vi "ALTS-2015 Decide Cases to go.vi"(8 "error in":errorcluster, 11 "DI Change Status":bool[](array[boolean])) -> (0 "error out":errorcluster, 2 "Station Selected":T1[](array[typedef]), 3 "Cases to go":string)   [LabVIEW 2013]
doc: "Copyright © 2005, Soliton Technologies.\nAll rights reserved."
uses:
  Controls/ALTS-2015 Station Cluster.ctl
  Controls/ALTS-2015 LV2GBL Options.ctl
  SLL DAQ Engine/Software/Source Code/Sub VIs/DAQ Engine/Controls/SLL DE List of Digital Inputs.ctl
  Controls/ALTS-2015 States.ctl
  Controls/ALTS-2015 Air Leak Test System-Main Screen Cases.ctl
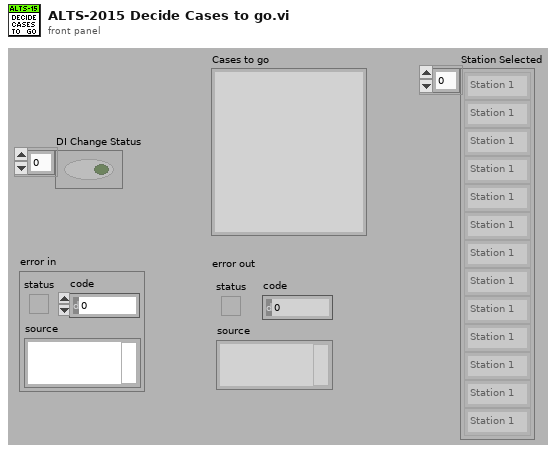
[diagram p1: front panel]
types:
  T1 = typedef "ALTS-2015 Station Cluster.ctl" = enum16{"Station 1", "Station 2", "Station 3", "Station 4"}
  T2 = typedef "ALTS-2015 LV2GBL Options.ctl" = enum16{"Read all", "Write all"}
  T3 = typedef "SLL DE List of Digital Inputs.ctl" = enum16{"STATION1_START", "STATION1_STOP", "STATION1_CLAMPED", "STATION1_TC_PASS", "STATION1_TC_FAIL", "STATION2_START", "STATION2_STOP", "STATION2_CLAMPED", "STATION2_TC_PASS", "STATION2_TC_FAIL", "STATION3_START", "STATION3_STOP", "STATION3_CLAMPED", "STATION3_TC_PASS", "STATION3_TC_FAIL", "STATION4_START", "STATION4_STOP", "STATION4_CLAMPED", "STATION4_TC_PASS", "STATION4_TC_FAIL"}
  T4 = typedef "ALTS-2015 Air Leak Test System-Main Screen Cases.ctl" = enum16{">PollEvents", ">Initialize", ">Exit", ">Error", ">EmptyCase", ">Get User Login", ">Initial FP update", ">Scan Serial Number", ">Check DI Status", ">Check for UUT Clamped & start Test", ">Stop the Test", ">Restore station after stop pressed", ">UUT Clamped", ">UUT Unclamped", ">Test Complete Failed", ">Read Test Data Result - Pass", ">Read Test Data Result - Fail", ">Write Result to DB", ">Update Station Info"}
  T5 = typedef "ALTS-2015 States.ctl" = enum16{"Initialize", "Poll", "Error", "Exit", "Authentication", "Scan Serial No", "Enqueue New Serial Task", "Enqueue Invalid Serial Task", "Enqueue Rerun Task", "Enqueu Unload Task", "Check DI Status", "Check UUT Clamp & Start Test", "Restore station after Stop Pressed", "Stop the Test", "UUT Clamped", "UUT Unclamped", "Test Complete Failed", "Read Test Data Result - Pass", "Read Test Data Result - Fail", "Write Result to DB", "Update Station Info"}
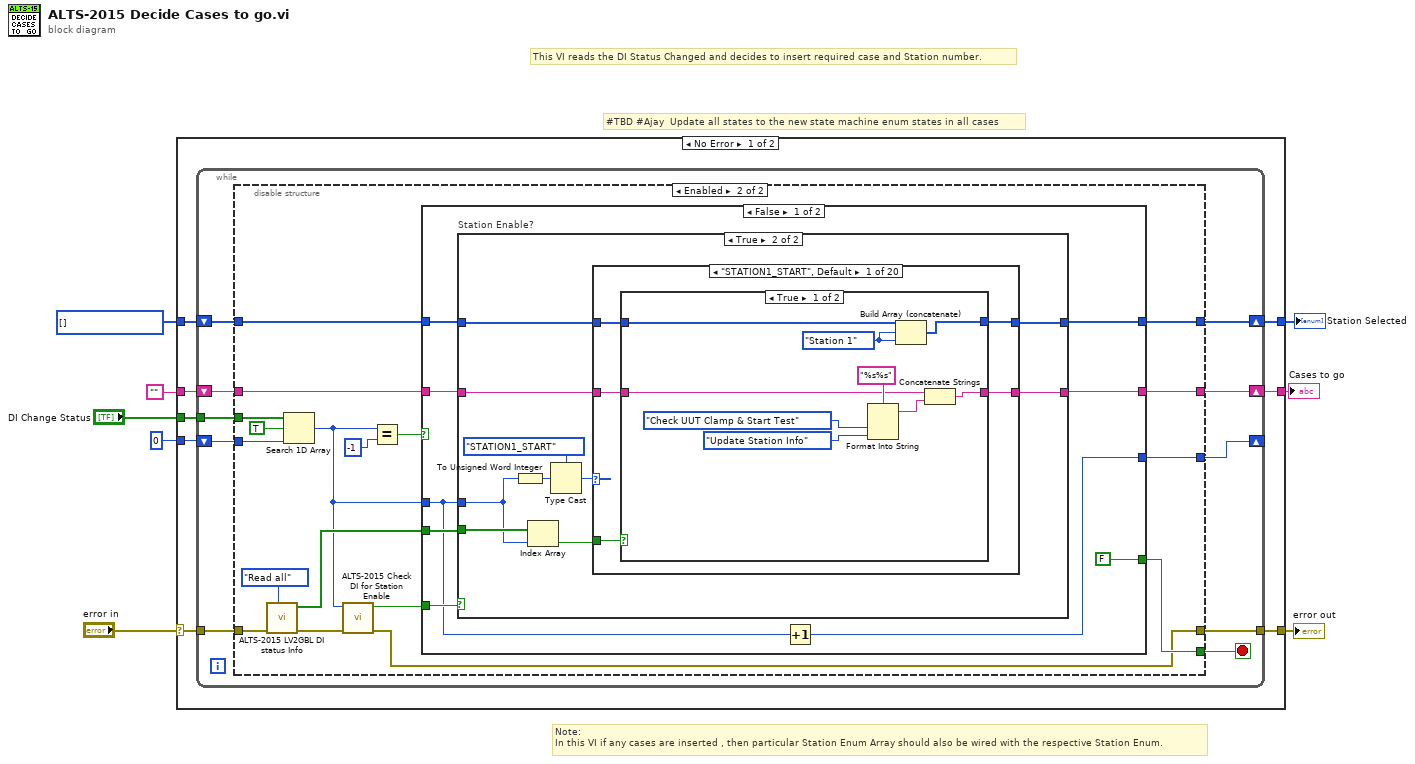
[diagram p0: block diagram]
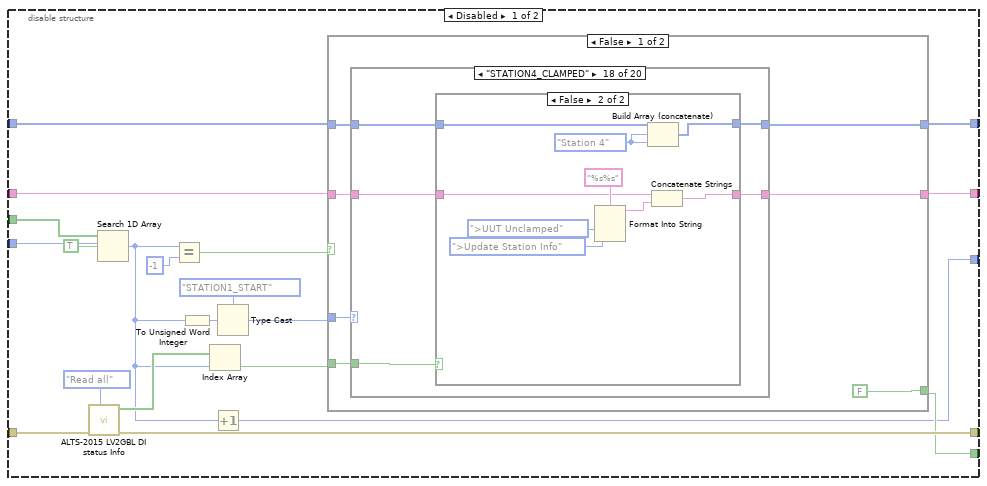
[diagram p2: hidden frame]
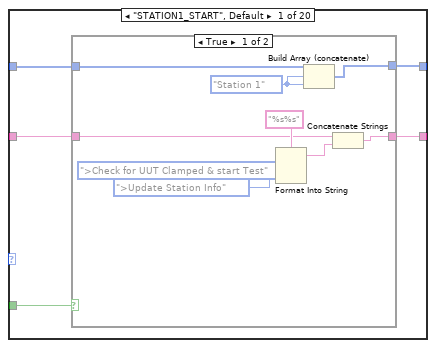
[diagram p3: hidden frame]
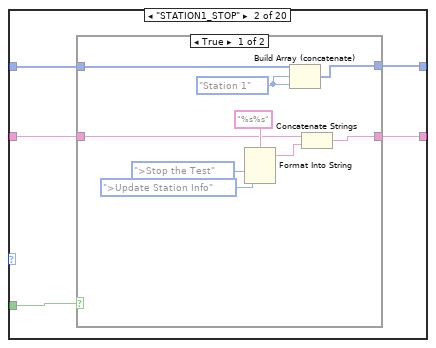
[diagram p5: hidden frame]
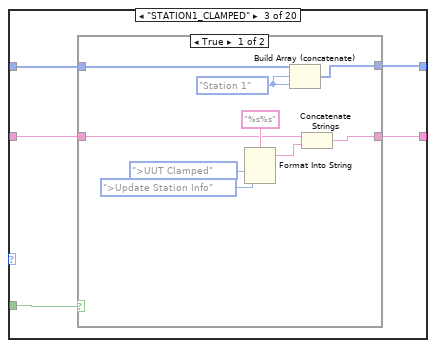
[diagram p7: hidden frame]
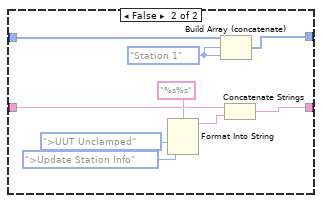
[diagram p8: hidden frame]
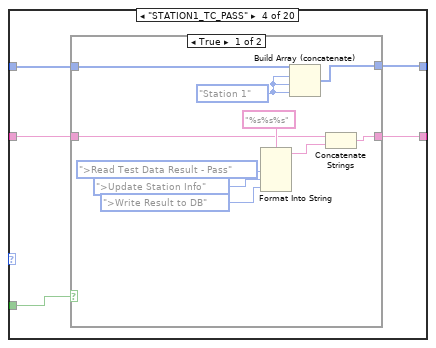
[diagram p9: hidden frame]
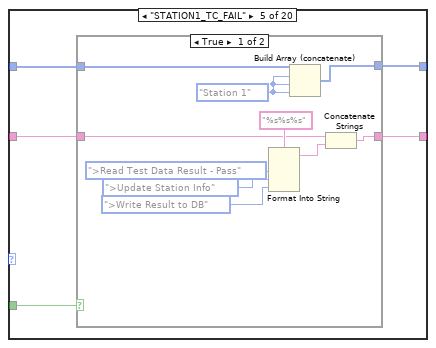
[diagram p11: hidden frame]
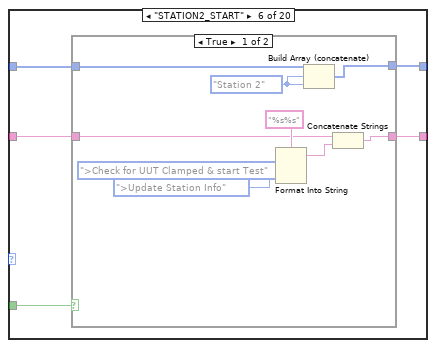
[diagram p13: hidden frame]
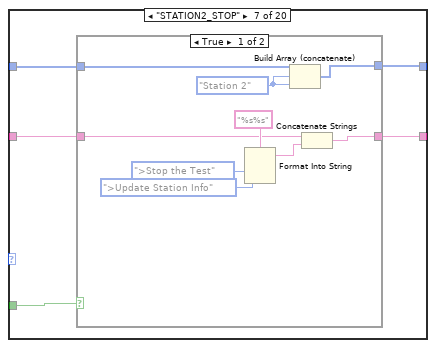
[diagram p15: hidden frame]
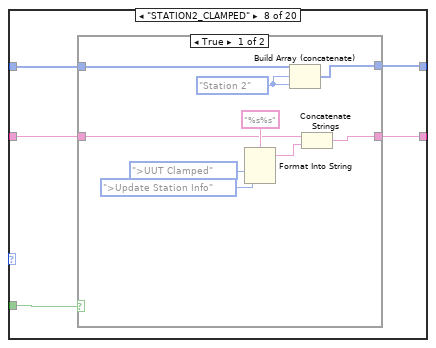
[diagram p17: hidden frame]
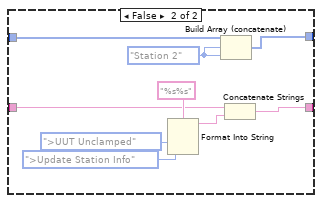
[diagram p18: hidden frame]
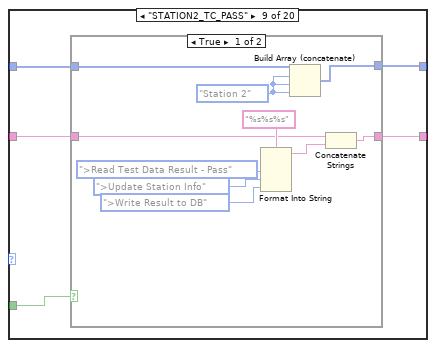
[diagram p19: hidden frame]
diagram:
  w3 = T1[] [] items=["Station 1", "Station 2", "Station 3", "Station 4"]
  # "#TBD #Ajay  Update all states to the new state machine enum states in all cases"
  # "Note: \nIn this VI if any cases are inserted , then particular Station Enum Array should also be wired with the respective Station Enum."
  # "This VI reads the DI Status Changed and decides to insert required case and Station number."
  n1 = case shown="No Error" "error in" {
    selector: "error in" -> [w14 w802]
    tunnel: [w13 w802] -> w8
    tunnel: "DI Change Status" -> [w10 _]
    tunnel: "" -> [w16 _]
    tunnel: [w15 ""] -> w4
    tunnel: w3 -> [w12 _]
    tunnel: [w11 w800] -> w2
    tunnel: 0 ("index of element") -> [w9 _]
    frame No Error {
      n2 = while {
        shift-right: [w20] -> w15
        shift-left: w16 -> [w26]
        tunnel: w14 -> [w25]
        tunnel: [w24] -> w13
        shift-right: [w22] -> w11
        shift-left: w12 -> [w23]
        tunnel: w10 -> [w19]
        shift-right: [w17] -> _
        shift-left: w9 -> [w18]
        stop <- w21 stop-if-true
        n3 = disable-structure shown="Enabled" {
          disable-tunnel: w26 -> [w41 w428]
          disable-tunnel: w25 -> [w39 w426]
          disable-tunnel: [w36 w413] -> w24
          disable-tunnel: w23 -> [w35 w424]
          disable-tunnel: [w34 w423] -> w22
          disable-tunnel: [w32 w422] -> w21
          disable-tunnel: [w31 w421] -> w20
          disable-tunnel: w19 -> [w30 w420]
          disable-tunnel: w18 -> [w28 w419]
          disable-tunnel: [w27 w418] -> w17
          frame Disabled {
            n4 = call "ALTS-2015 LV2GBL DI status Info.vi"("Options"=ALTS-2015_LV2GBL_Options."Read all", "error in"=w39) -> ("error out"=w36:errorcluster, "DI Status Out"=w38:bool[])  [unwired: 8 in]
            n5 = Search 1D Array(1D array=w30, element=TRUE, start index (0)=w28) -> (index of element=w29:i32)
            n6 = Equal?(x=w29, y=-1) -> (x = y?=w33:bool)
            n7 = To Unsigned Word Integer(number=w29) -> (unsigned 16bit integer=w43:u16)
            n8 = Index Array(array=w38, index=w29) -> (element=w37:bool)
            n9 = Increment(x=w29) -> (x+1=w27:i32)
            n10 = Type Cast(type=SLL_DE_List_of_Digital_Inputs."STATION1_START" ("DI Channel Name"), x=w43) -> (*(type *) &x=w42:T3)
            n11 = case shown="False" w33 {
              tunnel: w42 -> [w53 _]
              tunnel: w41 -> [w48 w411]
              tunnel: w37 -> [w52 _]
              tunnel: w35 -> [w51 w410]
              tunnel: [w50 w410] -> w34
              tunnel: [FALSE TRUE] -> w32
              tunnel: [w47 w411] -> w31
              frame False {
                n12 = case shown="\"STATION4_CLAMPED\"" w53 {
                  tunnel: w52 -> [w58 w74 w90 w113 w130 w147 w163 w179 w202 w219 w236 w252 w268 w291 w308 w325 w341 w357 w380 w397]
                  tunnel: w51 -> [w57 w73 w89 w112 w129 w146 w162 w178 w201 w218 w235 w251 w267 w290 w307 w324 w340 w356 w379 w396]
                  tunnel: [w56 w72 w88 w111 w128 w145 w161 w177 w200 w217 w234 w250 w266 w289 w306 w323 w339 w355 w378 w395] -> w50
                  tunnel: w48 -> [w55 w71 w87 w110 w127 w144 w160 w176 w199 w216 w233 w249 w265 w288 w305 w322 w338 w354 w377 w394]
                  tunnel: [w54 w70 w86 w109 w126 w143 w159 w175 w198 w215 w232 w248 w264 w287 w304 w321 w337 w353 w376 w393] -> w47
                  frame "STATION1_START", Default {
                    n13 = case shown="True" w58 {
                      tunnel: w57 -> [w65 w69]
                      tunnel: [w64 w69] -> w56
                      tunnel: w55 -> [w63 w68]
                      tunnel: [w61 w68] -> w54
                      frame True {
                        w59 = ALTS-2015_Station_Cluster."Station 1" ("Station Cluster")
                        n14 = Format Into String(format string="%s%s", ALTS-2015_Air_Leak_Test_System-Main_Screen_Cases.">Check for UUT Clamped & start Test" ("Cases"), ALTS-2015_Air_Leak_Test_System-Main_Screen_Cases.">Update Station Info" ("input 2")) -> (resulting string=w62:string)  [unwired: 2 in, 1 out]
                        n15 = Build Array (concatenate)(w65, w59, w59) -> (w64:T1[])
                        n16 = Concatenate Strings(w63, w62) -> (w61:string)
                      }
                      frame False {
                      }
                    }
                  }
                  frame "STATION1_STOP" {
                    n17 = case shown="True" w74 {
                      tunnel: w73 -> [w81 w85]
                      tunnel: [w80 w85] -> w72
                      tunnel: w71 -> [w79 w84]
                      tunnel: [w77 w84] -> w70
                      frame True {
                        w75 = ALTS-2015_Station_Cluster."Station 1" ("Station Cluster")
                        n18 = Format Into String(format string="%s%s", ALTS-2015_Air_Leak_Test_System-Main_Screen_Cases.">Stop the Test" ("Cases"), ALTS-2015_Air_Leak_Test_System-Main_Screen_Cases.">Update Station Info" ("input 2")) -> (resulting string=w78:string)  [unwired: 2 in, 1 out]
                        n19 = Build Array (concatenate)(w81, w75, w75) -> (w80:T1[])
                        n20 = Concatenate Strings(w79, w78) -> (w77:string)
                      }
                      frame False {
                      }
                    }
                  }
                  frame "STATION1_CLAMPED" {
                    n21 = case shown="True" w90 {
                      tunnel: w89 -> [w97 w106]
                      tunnel: [w96 w105] -> w88
                      tunnel: w87 -> [w95 w104]
                      tunnel: [w93 w102] -> w86
                      frame True {
                        w91 = ALTS-2015_Station_Cluster."Station 1" ("Station Cluster")
                        n22 = Format Into String(format string="%s%s", ALTS-2015_Air_Leak_Test_System-Main_Screen_Cases.">UUT Clamped" ("Cases"), ALTS-2015_Air_Leak_Test_System-Main_Screen_Cases.">Update Station Info" ("input 2")) -> (resulting string=w94:string)  [unwired: 2 in, 1 out]
                        n23 = Build Array (concatenate)(w97, w91, w91) -> (w96:T1[])
                        n24 = Concatenate Strings(w95, w94) -> (w93:string)
                      }
                      frame False {
                        w100 = ALTS-2015_Station_Cluster."Station 1" ("Station Cluster")
                        n25 = Format Into String(format string="%s%s", ALTS-2015_Air_Leak_Test_System-Main_Screen_Cases.">UUT Unclamped" ("Cases"), ALTS-2015_Air_Leak_Test_System-Main_Screen_Cases.">Update Station Info" ("input 2")) -> (resulting string=w103:string)  [unwired: 2 in, 1 out]
                        n26 = Build Array (concatenate)(w106, w100, w100) -> (w105:T1[])
                        n27 = Concatenate Strings(w104, w103) -> (w102:string)
                      }
                    }
                  }
                  frame "STATION1_TC_PASS" {
                    n28 = case shown="True" w113 {
                      tunnel: w112 -> [w121 w125]
                      tunnel: [w120 w125] -> w111
                      tunnel: w110 -> [w119 w124]
                      tunnel: [w117 w124] -> w109
                      frame True {
                        w114 = ALTS-2015_Station_Cluster."Station 1" ("Station Cluster")
                        n29 = Format Into String(format string="%s%s%s", ALTS-2015_Air_Leak_Test_System-Main_Screen_Cases.">Read Test Data Result - Pass" ("Cases"), ALTS-2015_Air_Leak_Test_System-Main_Screen_Cases.">Update Station Info" ("input 2"), ALTS-2015_Air_Leak_Test_System-Main_Screen_Cases.">Write Result to DB" ("input 2")) -> (resulting string=w118:string)  [unwired: 2 in, 1 out]
                        n30 = Build Array (concatenate)(w121, w114, w114, w114) -> (w120:T1[])
                        n31 = Concatenate Strings(w119, w118) -> (w117:string)
                      }
                      frame False {
                      }
                    }
                  }
                  frame "STATION1_TC_FAIL" {
                    n32 = case shown="True" w130 {
                      tunnel: w129 -> [w138 w142]
                      tunnel: [w137 w142] -> w128
                      tunnel: w127 -> [w136 w141]
                      tunnel: [w134 w141] -> w126
                      frame True {
                        w131 = ALTS-2015_Station_Cluster."Station 1" ("Station Cluster")
                        n33 = Format Into String(format string="%s%s%s", ALTS-2015_Air_Leak_Test_System-Main_Screen_Cases.">Read Test Data Result - Pass" ("Cases"), ALTS-2015_Air_Leak_Test_System-Main_Screen_Cases.">Update Station Info" ("input 2"), ALTS-2015_Air_Leak_Test_System-Main_Screen_Cases.">Write Result to DB" ("input 3")) -> (resulting string=w135:string)  [unwired: 2 in, 1 out]
                        n34 = Build Array (concatenate)(w138, w131, w131, w131) -> (w137:T1[])
                        n35 = Concatenate Strings(w136, w135) -> (w134:string)
                      }
                      frame False {
                      }
                    }
                  }
                  frame "STATION2_START" {
                    n36 = case shown="True" w147 {
                      tunnel: w146 -> [w154 w158]
                      tunnel: [w153 w158] -> w145
                      tunnel: w144 -> [w152 w157]
                      tunnel: [w150 w157] -> w143
                      frame True {
                        w148 = ALTS-2015_Station_Cluster."Station 2" ("Station Cluster")
                        n37 = Format Into String(format string="%s%s", ALTS-2015_Air_Leak_Test_System-Main_Screen_Cases.">Check for UUT Clamped & start Test" ("Cases"), ALTS-2015_Air_Leak_Test_System-Main_Screen_Cases.">Update Station Info" ("input 2")) -> (resulting string=w151:string)  [unwired: 2 in, 1 out]
                        n38 = Build Array (concatenate)(w154, w148, w148) -> (w153:T1[])
                        n39 = Concatenate Strings(w152, w151) -> (w150:string)
                      }
                      frame False {
                      }
                    }
                  }
                  frame "STATION2_STOP" {
                    n40 = case shown="True" w163 {
                      tunnel: w162 -> [w170 w174]
                      tunnel: [w169 w174] -> w161
                      tunnel: w160 -> [w168 w173]
                      tunnel: [w166 w173] -> w159
                      frame True {
                        w164 = ALTS-2015_Station_Cluster."Station 2" ("Station Cluster")
                        n41 = Format Into String(format string="%s%s", ALTS-2015_Air_Leak_Test_System-Main_Screen_Cases.">Stop the Test" ("Cases"), ALTS-2015_Air_Leak_Test_System-Main_Screen_Cases.">Update Station Info" ("input 2")) -> (resulting string=w167:string)  [unwired: 2 in, 1 out]
                        n42 = Build Array (concatenate)(w170, w164, w164) -> (w169:T1[])
                        n43 = Concatenate Strings(w168, w167) -> (w166:string)
                      }
                      frame False {
                      }
                    }
                  }
                  frame "STATION2_CLAMPED" {
                    n44 = case shown="True" w179 {
                      tunnel: w178 -> [w186 w195]
                      tunnel: [w185 w194] -> w177
                      tunnel: w176 -> [w184 w193]
                      tunnel: [w182 w191] -> w175
                      frame True {
                        w180 = ALTS-2015_Station_Cluster."Station 2" ("Station Cluster")
                        n45 = Format Into String(format string="%s%s", ALTS-2015_Air_Leak_Test_System-Main_Screen_Cases.">UUT Clamped" ("Cases"), ALTS-2015_Air_Leak_Test_System-Main_Screen_Cases.">Update Station Info" ("input 2")) -> (resulting string=w183:string)  [unwired: 2 in, 1 out]
                        n46 = Build Array (concatenate)(w186, w180, w180) -> (w185:T1[])
                        n47 = Concatenate Strings(w184, w183) -> (w182:string)
                      }
                      frame False {
                        w189 = ALTS-2015_Station_Cluster."Station 2" ("Station Cluster")
                        n48 = Format Into String(format string="%s%s", ALTS-2015_Air_Leak_Test_System-Main_Screen_Cases.">UUT Unclamped" ("Cases"), ALTS-2015_Air_Leak_Test_System-Main_Screen_Cases.">Update Station Info" ("input 2")) -> (resulting string=w192:string)  [unwired: 2 in, 1 out]
                        n49 = Build Array (concatenate)(w195, w189, w189) -> (w194:T1[])
                        n50 = Concatenate Strings(w193, w192) -> (w191:string)
                      }
                    }
                  }
                  frame "STATION2_TC_PASS" {
                    n51 = case shown="True" w202 {
                      tunnel: w201 -> [w210 w214]
                      tunnel: [w209 w214] -> w200
                      tunnel: w199 -> [w208 w213]
                      tunnel: [w206 w213] -> w198
                      frame True {
                        w203 = ALTS-2015_Station_Cluster."Station 2" ("Station Cluster")
                        n52 = Format Into String(format string="%s%s%s", ALTS-2015_Air_Leak_Test_System-Main_Screen_Cases.">Read Test Data Result - Pass" ("Cases"), ALTS-2015_Air_Leak_Test_System-Main_Screen_Cases.">Update Station Info" ("input 2"), ALTS-2015_Air_Leak_Test_System-Main_Screen_Cases.">Write Result to DB" ("input 2")) -> (resulting string=w207:string)  [unwired: 2 in, 1 out]
                        n53 = Build Array (concatenate)(w210, w203, w203, w203) -> (w209:T1[])
                        n54 = Concatenate Strings(w208, w207) -> (w206:string)
                      }
                      frame False {
                      }
                    }
                  }
                  frame "STATION2_TC_FAIL" {
                    n55 = case shown="True" w219 {
                      tunnel: w218 -> [w227 w231]
                      tunnel: [w226 w231] -> w217
                      tunnel: w216 -> [w225 w230]
                      tunnel: [w223 w230] -> w215
                      frame True {
                        w220 = ALTS-2015_Station_Cluster."Station 2" ("Station Cluster")
                        n56 = Format Into String(format string="%s%s%s", ALTS-2015_Air_Leak_Test_System-Main_Screen_Cases.">Read Test Data Result - Pass" ("Cases"), ALTS-2015_Air_Leak_Test_System-Main_Screen_Cases.">Update Station Info" ("input 2"), ALTS-2015_Air_Leak_Test_System-Main_Screen_Cases.">Write Result to DB" ("input 3")) -> (resulting string=w224:string)  [unwired: 2 in, 1 out]
                        n57 = Build Array (concatenate)(w227, w220, w220, w220) -> (w226:T1[])
                        n58 = Concatenate Strings(w225, w224) -> (w223:string)
                      }
                      frame False {
                      }
                    }
                  }
                  frame "STATION3_START" {
                    n59 = case shown="True" w236 {
                      tunnel: w235 -> [w243 w247]
                      tunnel: [w242 w247] -> w234
                      tunnel: w233 -> [w241 w246]
                      tunnel: [w239 w246] -> w232
                      frame True {
                        w237 = ALTS-2015_Station_Cluster."Station 3" ("Station Cluster")
                        n60 = Format Into String(format string="%s%s", ALTS-2015_Air_Leak_Test_System-Main_Screen_Cases.">Check for UUT Clamped & start Test" ("Cases"), ALTS-2015_Air_Leak_Test_System-Main_Screen_Cases.">Update Station Info" ("input 2")) -> (resulting string=w240:string)  [unwired: 2 in, 1 out]
                        n61 = Build Array (concatenate)(w243, w237, w237) -> (w242:T1[])
                        n62 = Concatenate Strings(w241, w240) -> (w239:string)
                      }
                      frame False {
                      }
                    }
                  }
                  frame "STATION3_STOP" {
                    n63 = case shown="True" w252 {
                      tunnel: w251 -> [w259 w263]
                      tunnel: [w258 w263] -> w250
                      tunnel: w249 -> [w257 w262]
                      tunnel: [w255 w262] -> w248
                      frame True {
                        w253 = ALTS-2015_Station_Cluster."Station 3" ("Station Cluster")
                        n64 = Format Into String(format string="%s%s", ALTS-2015_Air_Leak_Test_System-Main_Screen_Cases.">Stop the Test" ("Cases"), ALTS-2015_Air_Leak_Test_System-Main_Screen_Cases.">Update Station Info" ("input 2")) -> (resulting string=w256:string)  [unwired: 2 in, 1 out]
                        n65 = Build Array (concatenate)(w259, w253, w253) -> (w258:T1[])
                        n66 = Concatenate Strings(w257, w256) -> (w255:string)
                      }
                      frame False {
                      }
                    }
                  }
                  frame "STATION3_CLAMPED" {
                    n67 = case shown="False" w268 {
                      tunnel: w267 -> [w275 w284]
                      tunnel: [w274 w283] -> w266
                      tunnel: w265 -> [w273 w282]
                      tunnel: [w271 w280] -> w264
                      frame True {
                        w269 = ALTS-2015_Station_Cluster."Station 3" ("Station Cluster")
                        n68 = Format Into String(format string="%s%s", ALTS-2015_Air_Leak_Test_System-Main_Screen_Cases.">UUT Clamped" ("Cases"), ALTS-2015_Air_Leak_Test_System-Main_Screen_Cases.">Update Station Info" ("input 2")) -> (resulting string=w272:string)  [unwired: 2 in, 1 out]
                        n69 = Build Array (concatenate)(w275, w269, w269) -> (w274:T1[])
                        n70 = Concatenate Strings(w273, w272) -> (w271:string)
                      }
                      frame False {
                        w278 = ALTS-2015_Station_Cluster."Station 3" ("Station Cluster")
                        n71 = Format Into String(format string="%s%s", ALTS-2015_Air_Leak_Test_System-Main_Screen_Cases.">UUT Unclamped" ("Cases"), ALTS-2015_Air_Leak_Test_System-Main_Screen_Cases.">Update Station Info" ("input 2")) -> (resulting string=w281:string)  [unwired: 2 in, 1 out]
                        n72 = Build Array (concatenate)(w284, w278, w278) -> (w283:T1[])
                        n73 = Concatenate Strings(w282, w281) -> (w280:string)
                      }
                    }
                  }
                  frame "STATION3_TC_PASS" {
                    n74 = case shown="True" w291 {
                      tunnel: w290 -> [w299 w303]
                      tunnel: [w298 w303] -> w289
                      tunnel: w288 -> [w297 w302]
                      tunnel: [w295 w302] -> w287
                      frame True {
                        w292 = ALTS-2015_Station_Cluster."Station 3" ("Station Cluster")
                        n75 = Format Into String(format string="%s%s%s", ALTS-2015_Air_Leak_Test_System-Main_Screen_Cases.">Read Test Data Result - Pass" ("Cases"), ALTS-2015_Air_Leak_Test_System-Main_Screen_Cases.">Update Station Info" ("input 2"), ALTS-2015_Air_Leak_Test_System-Main_Screen_Cases.">Write Result to DB" ("input 2")) -> (resulting string=w296:string)  [unwired: 2 in, 1 out]
                        n76 = Build Array (concatenate)(w299, w292, w292, w292) -> (w298:T1[])
                        n77 = Concatenate Strings(w297, w296) -> (w295:string)
                      }
                      frame False {
                      }
                    }
                  }
                  frame "STATION3_TC_FAIL" {
                    n78 = case shown="True" w308 {
                      tunnel: w307 -> [w316 w320]
                      tunnel: [w315 w320] -> w306
                      tunnel: w305 -> [w314 w319]
                      tunnel: [w312 w319] -> w304
                      frame True {
                        w309 = ALTS-2015_Station_Cluster."Station 3" ("Station Cluster")
                        n79 = Format Into String(format string="%s%s%s", ALTS-2015_Air_Leak_Test_System-Main_Screen_Cases.">Read Test Data Result - Pass" ("Cases"), ALTS-2015_Air_Leak_Test_System-Main_Screen_Cases.">Update Station Info" ("input 2"), ALTS-2015_Air_Leak_Test_System-Main_Screen_Cases.">Write Result to DB" ("input 3")) -> (resulting string=w313:string)  [unwired: 2 in, 1 out]
                        n80 = Build Array (concatenate)(w316, w309, w309, w309) -> (w315:T1[])
                        n81 = Concatenate Strings(w314, w313) -> (w312:string)
                      }
                      frame False {
                      }
                    }
                  }
                  frame "STATION4_START" {
                    n82 = case shown="True" w325 {
                      tunnel: w324 -> [w332 w336]
                      tunnel: [w331 w336] -> w323
                      tunnel: w322 -> [w330 w335]
                      tunnel: [w328 w335] -> w321
                      frame True {
                        w326 = ALTS-2015_Station_Cluster."Station 4" ("Station Cluster")
                        n83 = Format Into String(format string="%s%s", ALTS-2015_Air_Leak_Test_System-Main_Screen_Cases.">Check for UUT Clamped & start Test" ("Cases"), ALTS-2015_Air_Leak_Test_System-Main_Screen_Cases.">Update Station Info" ("input 2")) -> (resulting string=w329:string)  [unwired: 2 in, 1 out]
                        n84 = Build Array (concatenate)(w332, w326, w326) -> (w331:T1[])
                        n85 = Concatenate Strings(w330, w329) -> (w328:string)
                      }
                      frame False {
                      }
                    }
                  }
                  frame "STATION4_STOP" {
                    n86 = case shown="True" w341 {
                      tunnel: w340 -> [w348 w352]
                      tunnel: [w347 w352] -> w339
                      tunnel: w338 -> [w346 w351]
                      tunnel: [w344 w351] -> w337
                      frame True {
                        w342 = ALTS-2015_Station_Cluster."Station 4" ("Station Cluster")
                        n87 = Format Into String(format string="%s%s", ALTS-2015_Air_Leak_Test_System-Main_Screen_Cases.">Stop the Test" ("Cases"), ALTS-2015_Air_Leak_Test_System-Main_Screen_Cases.">Update Station Info" ("input 2")) -> (resulting string=w345:string)  [unwired: 2 in, 1 out]
                        n88 = Build Array (concatenate)(w348, w342, w342) -> (w347:T1[])
                        n89 = Concatenate Strings(w346, w345) -> (w344:string)
                      }
                      frame False {
                      }
                    }
                  }
                  frame "STATION4_CLAMPED" {
                    n90 = case shown="False" w357 {
                      tunnel: w356 -> [w364 w373]
                      tunnel: [w363 w372] -> w355
                      tunnel: w354 -> [w362 w371]
                      tunnel: [w360 w369] -> w353
                      frame True {
                        w358 = ALTS-2015_Station_Cluster."Station 4" ("Station Cluster")
                        n91 = Format Into String(format string="%s%s", ALTS-2015_Air_Leak_Test_System-Main_Screen_Cases.">UUT Clamped" ("Cases"), ALTS-2015_Air_Leak_Test_System-Main_Screen_Cases.">Update Station Info" ("input 2")) -> (resulting string=w361:string)  [unwired: 2 in, 1 out]
                        n92 = Build Array (concatenate)(w364, w358, w358) -> (w363:T1[])
                        n93 = Concatenate Strings(w362, w361) -> (w360:string)
                      }
                      frame False {
                        w367 = ALTS-2015_Station_Cluster."Station 4" ("Station Cluster")
                        n94 = Format Into String(format string="%s%s", ALTS-2015_Air_Leak_Test_System-Main_Screen_Cases.">UUT Unclamped" ("Cases"), ALTS-2015_Air_Leak_Test_System-Main_Screen_Cases.">Update Station Info" ("input 2")) -> (resulting string=w370:string)  [unwired: 2 in, 1 out]
                        n95 = Build Array (concatenate)(w373, w367, w367) -> (w372:T1[])
                        n96 = Concatenate Strings(w371, w370) -> (w369:string)
                      }
                    }
                  }
                  frame "STATION4_TC_PASS" {
                    n97 = case shown="True" w380 {
                      tunnel: w379 -> [w388 w392]
                      tunnel: [w387 w392] -> w378
                      tunnel: w377 -> [w386 w391]
                      tunnel: [w384 w391] -> w376
                      frame True {
                        w381 = ALTS-2015_Station_Cluster."Station 4" ("Station Cluster")
                        n98 = Format Into String(format string="%s%s%s", ALTS-2015_Air_Leak_Test_System-Main_Screen_Cases.">Read Test Data Result - Pass" ("Cases"), ALTS-2015_Air_Leak_Test_System-Main_Screen_Cases.">Update Station Info" ("input 2"), ALTS-2015_Air_Leak_Test_System-Main_Screen_Cases.">Write Result to DB" ("input 2")) -> (resulting string=w385:string)  [unwired: 2 in, 1 out]
                        n99 = Build Array (concatenate)(w388, w381, w381, w381) -> (w387:T1[])
                        n100 = Concatenate Strings(w386, w385) -> (w384:string)
                      }
                      frame False {
                      }
                    }
                  }
                  frame "STATION4_TC_FAIL" {
                    n101 = case shown="True" w397 {
                      tunnel: w396 -> [w405 w409]
                      tunnel: [w404 w409] -> w395
                      tunnel: w394 -> [w403 w408]
                      tunnel: [w401 w408] -> w393
                      frame True {
                        w398 = ALTS-2015_Station_Cluster."Station 4" ("Station Cluster")
                        n102 = Format Into String(format string="%s%s%s", ALTS-2015_Air_Leak_Test_System-Main_Screen_Cases.">Read Test Data Result - Pass" ("Cases"), ALTS-2015_Air_Leak_Test_System-Main_Screen_Cases.">Update Station Info" ("input 2"), ALTS-2015_Air_Leak_Test_System-Main_Screen_Cases.">Write Result to DB" ("input 3")) -> (resulting string=w402:string)  [unwired: 2 in, 1 out]
                        n103 = Build Array (concatenate)(w405, w398, w398, w398) -> (w404:T1[])
                        n104 = Concatenate Strings(w403, w402) -> (w401:string)
                      }
                      frame False {
                      }
                    }
                  }
                }
              }
              frame True {
              }
            }
          }
          frame Enabled {
            n105 = call "ALTS-2015 LV2GBL DI status Info.vi"("Options"=ALTS-2015_LV2GBL_Options."Read all", "error in"=w426) -> ("error out"=w416:errorcluster, "DI Status Out"=w425:bool[])  [unwired: 8 in]
            n106 = Search 1D Array(1D array=w420, element=TRUE, start index (0)=w419) -> (index of element=w417:i32)
            n107 = call "ALTS-2015 Check DI for Station Enable.vi"("error in"=w416, "DI Index"=w417) -> ("error out"=w413:errorcluster, "Station Enable?"=w414:bool)  [unwired: 8 in]
            n108 = Equal?(x=w417, y=-1) -> (x = y?=w415:bool)
            n109 = case shown="False" w415 {
              tunnel: w428 -> [w439 w797]
              tunnel: w425 -> [w434 _]
              tunnel: w424 -> [w438 w798]
              tunnel: [w437 w798] -> w423
              tunnel: w414 -> [w436 _]
              tunnel: [FALSE TRUE] -> w422
              tunnel: [w435 w797] -> w421
              tunnel: [w431 w796] -> w418
              tunnel: w417 -> [w432 w796]
              frame False {
                n110 = case "Station Enable?" shown="True" w436 {
                  tunnel: w439 -> [w441 w449]
                  tunnel: w438 -> [w440 w451]
                  tunnel: [w440 w450] -> w437
                  tunnel: [w441 w448] -> w435
                  tunnel: w434 -> [_ w446]
                  tunnel: w432 -> [_ w445]
                  frame False {
                  }
                  frame True {
                    n111 = To Unsigned Word Integer(number=w445) -> (unsigned 16bit integer=w447:u16)
                    n112 = Index Array(array=w446, index=w445) -> (element=w444:bool)
                    n113 = Type Cast(type=SLL_DE_List_of_Digital_Inputs."STATION1_START" ("DI Channel Name"), x=w447) -> (*(type *) &x=w442:T3)
                    n114 = case shown="\"STATION1_START\", Default" w442 {
                      tunnel: w444 -> [w456 w472 w489 w512 w527 w542 w558 w575 w598 w613 w628 w644 w661 w684 w699 w714 w730 w747 w770 w785]
                      tunnel: w451 -> [w455 w471 w488 w511 w526 w541 w557 w574 w597 w612 w627 w643 w660 w683 w698 w713 w729 w746 w769 w784]
                      tunnel: [w454 w470 w487 w510 w525 w540 w556 w573 w596 w611 w626 w642 w659 w682 w697 w712 w728 w745 w768 w783] -> w450
                      tunnel: w449 -> [w453 w469 w486 w509 w524 w539 w555 w572 w595 w610 w625 w641 w658 w681 w696 w711 w727 w744 w767 w782]
                      tunnel: [w452 w468 w485 w508 w523 w538 w554 w571 w594 w609 w624 w640 w657 w680 w695 w710 w726 w743 w766 w781] -> w448
                      frame "STATION1_START", Default {
                        n115 = case shown="True" w456 {
                          tunnel: w455 -> [w464 w467]
                          tunnel: [w463 w467] -> w454
                          tunnel: w453 -> [w462 w466]
                          tunnel: [w460 w466] -> w452
                          frame True {
                            w459 = ALTS-2015_Station_Cluster."Station 1" ("Station Cluster")
                            n116 = Format Into String(format string="%s%s", ALTS-2015_States."Check UUT Clamp & Start Test", ALTS-2015_States."Update Station Info") -> (resulting string=w461:string)  [unwired: 2 in, 1 out]
                            n117 = Build Array (concatenate)(w464, w459, w459) -> (w463:T1[])
                            n118 = Concatenate Strings(w462, w461) -> (w460:string)
                          }
                          frame False {
                          }
                        }
                      }
                      frame "STATION1_STOP" {
                        n119 = case shown="True" w472 {
                          tunnel: w471 -> [w481 w484]
                          tunnel: [w480 w484] -> w470
                          tunnel: w469 -> [w479 w483]
                          tunnel: [w477 w483] -> w468
                          frame True {
                            w476 = ALTS-2015_Station_Cluster."Station 1" ("Station Cluster")
                            n120 = Format Into String(format string="%s%s%s", ALTS-2015_States."Stop the Test", ALTS-2015_States."Restore station after Stop Pressed", ALTS-2015_States."Update Station Info") -> (resulting string=w478:string)  [unwired: 2 in, 1 out]
                            n121 = Build Array (concatenate)(w481, w476, w476, w476) -> (w480:T1[])
                            n122 = Concatenate Strings(w479, w478) -> (w477:string)
                          }
                          frame False {
                          }
                        }
                      }
                      frame "STATION1_CLAMPED" {
                        n123 = case shown="False" w489 {
                          tunnel: w488 -> [w497 w506]
                          tunnel: [w496 w505] -> w487
                          tunnel: w486 -> [w495 w504]
                          tunnel: [w493 w502] -> w485
                          frame True {
                            w492 = ALTS-2015_Station_Cluster."Station 1" ("Station Cluster")
                            n124 = Format Into String(format string="%s%s", ALTS-2015_States."UUT Clamped", ALTS-2015_States."Update Station Info") -> (resulting string=w494:string)  [unwired: 2 in, 1 out]
                            n125 = Build Array (concatenate)(w497, w492, w492) -> (w496:T1[])
                            n126 = Concatenate Strings(w495, w494) -> (w493:string)
                          }
                          frame False {
                            w501 = ALTS-2015_Station_Cluster."Station 1" ("Station Cluster")
                            n127 = Format Into String(format string="%s%s", ALTS-2015_States."UUT Unclamped", ALTS-2015_States."Update Station Info") -> (resulting string=w503:string)  [unwired: 2 in, 1 out]
                            n128 = Build Array (concatenate)(w506, w501, w501) -> (w505:T1[])
                            n129 = Concatenate Strings(w504, w503) -> (w502:string)
                          }
                        }
                      }
                      frame "STATION1_TC_PASS" {
                        n130 = case shown="True" w512 {
                          tunnel: w511 -> [w519 w522]
                          tunnel: [w518 w522] -> w510
                          tunnel: w509 -> [w517 w521]
                          tunnel: [w515 w521] -> w508
                          frame True {
                            n131 = Format Into String(format string="%s", ALTS-2015_States."Read Test Data Result - Pass") -> (resulting string=w516:string)  [unwired: 2 in, 1 out]
                            n132 = Build Array (concatenate)(w519, ALTS-2015_Station_Cluster."Station 1" ("Station Cluster")) -> (w518:T1[])
                            n133 = Concatenate Strings(w517, w516) -> (w515:string)
                          }
                          frame False {
                          }
                        }
                      }
                      frame "STATION1_TC_FAIL" {
                        n134 = case shown="True" w527 {
                          tunnel: w526 -> [w534 w537]
                          tunnel: [w533 w537] -> w525
                          tunnel: w524 -> [w532 w536]
                          tunnel: [w530 w536] -> w523
                          frame True {
                            n135 = Format Into String(format string="%s", ALTS-2015_States."Test Complete Failed") -> (resulting string=w531:string)  [unwired: 2 in, 1 out]
                            n136 = Build Array (concatenate)(w534, ALTS-2015_Station_Cluster."Station 1" ("Station Cluster")) -> (w533:T1[])
                            n137 = Concatenate Strings(w532, w531) -> (w530:string)
                          }
                          frame False {
                          }
                        }
                      }
                      frame "STATION2_START" {
                        n138 = case shown="True" w542 {
                          tunnel: w541 -> [w550 w553]
                          tunnel: [w549 w553] -> w540
                          tunnel: w539 -> [w548 w552]
                          tunnel: [w546 w552] -> w538
                          frame True {
                            w545 = ALTS-2015_Station_Cluster."Station 2" ("Station Cluster")
                            n139 = Format Into String(format string="%s%s", ALTS-2015_States."Check UUT Clamp & Start Test", ALTS-2015_States."Update Station Info") -> (resulting string=w547:string)  [unwired: 2 in, 1 out]
                            n140 = Build Array (concatenate)(w550, w545, w545) -> (w549:T1[])
                            n141 = Concatenate Strings(w548, w547) -> (w546:string)
                          }
                          frame False {
                          }
                        }
                      }
                      frame "STATION2_STOP" {
                        n142 = case shown="True" w558 {
                          tunnel: w557 -> [w567 w570]
                          tunnel: [w566 w570] -> w556
                          tunnel: w555 -> [w565 w569]
                          tunnel: [w563 w569] -> w554
                          frame True {
                            w562 = ALTS-2015_Station_Cluster."Station 2" ("Station Cluster")
                            n143 = Format Into String(format string="%s%s%s", ALTS-2015_States."Stop the Test", ALTS-2015_States."Restore station after Stop Pressed", ALTS-2015_States."Update Station Info") -> (resulting string=w564:string)  [unwired: 2 in, 1 out]
                            n144 = Build Array (concatenate)(w567, w562, w562, w562) -> (w566:T1[])
                            n145 = Concatenate Strings(w565, w564) -> (w563:string)
                          }
                          frame False {
                          }
                        }
                      }
                      frame "STATION2_CLAMPED" {
                        n146 = case shown="True" w575 {
                          tunnel: w574 -> [w583 w592]
                          tunnel: [w582 w591] -> w573
                          tunnel: w572 -> [w581 w590]
                          tunnel: [w579 w588] -> w571
                          frame True {
                            w578 = ALTS-2015_Station_Cluster."Station 2" ("Station Cluster")
                            n147 = Format Into String(format string="%s%s", ALTS-2015_States."UUT Clamped", ALTS-2015_States."Update Station Info") -> (resulting string=w580:string)  [unwired: 2 in, 1 out]
                            n148 = Build Array (concatenate)(w583, w578, w578) -> (w582:T1[])
                            n149 = Concatenate Strings(w581, w580) -> (w579:string)
                          }
                          frame False {
                            w587 = ALTS-2015_Station_Cluster."Station 2" ("Station Cluster")
                            n150 = Format Into String(format string="%s%s", ALTS-2015_States."UUT Unclamped", ALTS-2015_States."Update Station Info") -> (resulting string=w589:string)  [unwired: 2 in, 1 out]
                            n151 = Build Array (concatenate)(w592, w587, w587) -> (w591:T1[])
                            n152 = Concatenate Strings(w590, w589) -> (w588:string)
                          }
                        }
                      }
                      frame "STATION2_TC_PASS" {
                        n153 = case shown="True" w598 {
                          tunnel: w597 -> [w605 w608]
                          tunnel: [w604 w608] -> w596
                          tunnel: w595 -> [w603 w607]
                          tunnel: [w601 w607] -> w594
                          frame True {
                            n154 = Format Into String(format string="%s", ALTS-2015_States."Read Test Data Result - Pass") -> (resulting string=w602:string)  [unwired: 2 in, 1 out]
                            n155 = Build Array (concatenate)(w605, ALTS-2015_Station_Cluster."Station 2" ("Station Cluster")) -> (w604:T1[])
                            n156 = Concatenate Strings(w603, w602) -> (w601:string)
                          }
                          frame False {
                          }
                        }
                      }
                      frame "STATION2_TC_FAIL" {
                        n157 = case shown="True" w613 {
                          tunnel: w612 -> [w620 w623]
                          tunnel: [w619 w623] -> w611
                          tunnel: w610 -> [w618 w622]
                          tunnel: [w616 w622] -> w609
                          frame True {
                            n158 = Format Into String(format string="%s", ALTS-2015_States."Test Complete Failed") -> (resulting string=w617:string)  [unwired: 2 in, 1 out]
                            n159 = Build Array (concatenate)(w620, ALTS-2015_Station_Cluster."Station 2" ("Station Cluster")) -> (w619:T1[])
                            n160 = Concatenate Strings(w618, w617) -> (w616:string)
                          }
                          frame False {
                          }
                        }
                      }
                      frame "STATION3_START" {
                        n161 = case shown="True" w628 {
                          tunnel: w627 -> [w636 w639]
                          tunnel: [w635 w639] -> w626
                          tunnel: w625 -> [w634 w638]
                          tunnel: [w632 w638] -> w624
                          frame True {
                            w631 = ALTS-2015_Station_Cluster."Station 3" ("Station Cluster")
                            n162 = Format Into String(format string="%s%s", ALTS-2015_States."Check UUT Clamp & Start Test", ALTS-2015_States."Update Station Info") -> (resulting string=w633:string)  [unwired: 2 in, 1 out]
                            n163 = Build Array (concatenate)(w636, w631, w631) -> (w635:T1[])
                            n164 = Concatenate Strings(w634, w633) -> (w632:string)
                          }
                          frame False {
                          }
                        }
                      }
                      frame "STATION3_STOP" {
                        n165 = case shown="True" w644 {
                          tunnel: w643 -> [w653 w656]
                          tunnel: [w652 w656] -> w642
                          tunnel: w641 -> [w651 w655]
                          tunnel: [w649 w655] -> w640
                          frame True {
                            w648 = ALTS-2015_Station_Cluster."Station 3" ("Station Cluster")
                            n166 = Format Into String(format string="%s%s%s", ALTS-2015_States."Stop the Test", ALTS-2015_States."Restore station after Stop Pressed", ALTS-2015_States."Update Station Info") -> (resulting string=w650:string)  [unwired: 2 in, 1 out]
                            n167 = Build Array (concatenate)(w653, w648, w648, w648) -> (w652:T1[])
                            n168 = Concatenate Strings(w651, w650) -> (w649:string)
                          }
                          frame False {
                          }
                        }
                      }
                      frame "STATION3_CLAMPED" {
                        n169 = case shown="True" w661 {
                          tunnel: w660 -> [w669 w678]
                          tunnel: [w668 w677] -> w659
                          tunnel: w658 -> [w667 w676]
                          tunnel: [w665 w674] -> w657
                          frame True {
                            w664 = ALTS-2015_Station_Cluster."Station 3" ("Station Cluster")
                            n170 = Format Into String(format string="%s%s", ALTS-2015_States."UUT Clamped", ALTS-2015_States."Update Station Info") -> (resulting string=w666:string)  [unwired: 2 in, 1 out]
                            n171 = Build Array (concatenate)(w669, w664, w664) -> (w668:T1[])
                            n172 = Concatenate Strings(w667, w666) -> (w665:string)
                          }
                          frame False {
                            w673 = ALTS-2015_Station_Cluster."Station 3" ("Station Cluster")
                            n173 = Format Into String(format string="%s%s", ALTS-2015_States."UUT Unclamped", ALTS-2015_States."Update Station Info") -> (resulting string=w675:string)  [unwired: 2 in, 1 out]
                            n174 = Build Array (concatenate)(w678, w673, w673) -> (w677:T1[])
                            n175 = Concatenate Strings(w676, w675) -> (w674:string)
                          }
                        }
                      }
                      frame "STATION3_TC_PASS" {
                        n176 = case shown="True" w684 {
                          tunnel: w683 -> [w691 w694]
                          tunnel: [w690 w694] -> w682
                          tunnel: w681 -> [w689 w693]
                          tunnel: [w687 w693] -> w680
                          frame True {
                            n177 = Format Into String(format string="%s", ALTS-2015_States."Read Test Data Result - Pass") -> (resulting string=w688:string)  [unwired: 2 in, 1 out]
                            n178 = Build Array (concatenate)(w691, ALTS-2015_Station_Cluster."Station 3" ("Station Cluster")) -> (w690:T1[])
                            n179 = Concatenate Strings(w689, w688) -> (w687:string)
                          }
                          frame False {
                          }
                        }
                      }
                      frame "STATION3_TC_FAIL" {
                        n180 = case shown="True" w699 {
                          tunnel: w698 -> [w706 w709]
                          tunnel: [w705 w709] -> w697
                          tunnel: w696 -> [w704 w708]
                          tunnel: [w702 w708] -> w695
                          frame True {
                            n181 = Format Into String(format string="%s", ALTS-2015_States."Test Complete Failed") -> (resulting string=w703:string)  [unwired: 2 in, 1 out]
                            n182 = Build Array (concatenate)(w706, ALTS-2015_Station_Cluster."Station 3" ("Station Cluster")) -> (w705:T1[])
                            n183 = Concatenate Strings(w704, w703) -> (w702:string)
                          }
                          frame False {
                          }
                        }
                      }
                      frame "STATION4_START" {
                        n184 = case shown="True" w714 {
                          tunnel: w713 -> [w722 w725]
                          tunnel: [w721 w725] -> w712
                          tunnel: w711 -> [w720 w724]
                          tunnel: [w718 w724] -> w710
                          frame True {
                            w717 = ALTS-2015_Station_Cluster."Station 4" ("Station Cluster")
                            n185 = Format Into String(format string="%s%s", ALTS-2015_States."Check UUT Clamp & Start Test", ALTS-2015_States."Update Station Info") -> (resulting string=w719:string)  [unwired: 2 in, 1 out]
                            n186 = Build Array (concatenate)(w722, w717, w717) -> (w721:T1[])
                            n187 = Concatenate Strings(w720, w719) -> (w718:string)
                          }
                          frame False {
                          }
                        }
                      }
                      frame "STATION4_STOP" {
                        n188 = case shown="True" w730 {
                          tunnel: w729 -> [w739 w742]
                          tunnel: [w738 w742] -> w728
                          tunnel: w727 -> [w737 w741]
                          tunnel: [w735 w741] -> w726
                          frame True {
                            w734 = ALTS-2015_Station_Cluster."Station 4" ("Station Cluster")
                            n189 = Format Into String(format string="%s%s%s", ALTS-2015_States."Stop the Test", ALTS-2015_States."Restore station after Stop Pressed", ALTS-2015_States."Update Station Info") -> (resulting string=w736:string)  [unwired: 2 in, 1 out]
                            n190 = Build Array (concatenate)(w739, w734, w734, w734) -> (w738:T1[])
                            n191 = Concatenate Strings(w737, w736) -> (w735:string)
                          }
                          frame False {
                          }
                        }
                      }
                      frame "STATION4_CLAMPED" {
                        n192 = case shown="True" w747 {
                          tunnel: w746 -> [w755 w764]
                          tunnel: [w754 w763] -> w745
                          tunnel: w744 -> [w753 w762]
                          tunnel: [w751 w760] -> w743
                          frame True {
                            w750 = ALTS-2015_Station_Cluster."Station 4" ("Station Cluster")
                            n193 = Format Into String(format string="%s%s", ALTS-2015_States."UUT Clamped", ALTS-2015_States."Update Station Info") -> (resulting string=w752:string)  [unwired: 2 in, 1 out]
                            n194 = Build Array (concatenate)(w755, w750, w750) -> (w754:T1[])
                            n195 = Concatenate Strings(w753, w752) -> (w751:string)
                          }
                          frame False {
                            w759 = ALTS-2015_Station_Cluster."Station 4" ("Station Cluster")
                            n196 = Format Into String(format string="%s%s", ALTS-2015_States."UUT Unclamped", ALTS-2015_States."Update Station Info") -> (resulting string=w761:string)  [unwired: 2 in, 1 out]
                            n197 = Build Array (concatenate)(w764, w759, w759) -> (w763:T1[])
                            n198 = Concatenate Strings(w762, w761) -> (w760:string)
                          }
                        }
                      }
                      frame "STATION4_TC_PASS" {
                        n199 = case shown="True" w770 {
                          tunnel: w769 -> [w777 w780]
                          tunnel: [w776 w780] -> w768
                          tunnel: w767 -> [w775 w779]
                          tunnel: [w773 w779] -> w766
                          frame True {
                            n200 = Format Into String(format string="%s", ALTS-2015_States."Read Test Data Result - Pass") -> (resulting string=w774:string)  [unwired: 2 in, 1 out]
                            n201 = Build Array (concatenate)(w777, ALTS-2015_Station_Cluster."Station 4" ("Station Cluster")) -> (w776:T1[])
                            n202 = Concatenate Strings(w775, w774) -> (w773:string)
                          }
                          frame False {
                          }
                        }
                      }
                      frame "STATION4_TC_FAIL" {
                        n203 = case shown="True" w785 {
                          tunnel: w784 -> [w792 w795]
                          tunnel: [w791 w795] -> w783
                          tunnel: w782 -> [w790 w794]
                          tunnel: [w788 w794] -> w781
                          frame True {
                            n204 = Format Into String(format string="%s", ALTS-2015_States."Test Complete Failed") -> (resulting string=w789:string)  [unwired: 2 in, 1 out]
                            n205 = Build Array (concatenate)(w792, ALTS-2015_Station_Cluster."Station 4" ("Station Cluster")) -> (w791:T1[])
                            n206 = Concatenate Strings(w790, w789) -> (w788:string)
                          }
                          frame False {
                          }
                        }
                      }
                    }
                  }
                }
                n207 = Increment(x=w432) -> (x+1=w431:i32)
              }
              frame True {
              }
            }
          }
        }
      }
    }
    frame Error {
      w800 = T1[] [] items=["Station 1", "Station 2", "Station 3", "Station 4"]
    }
  }
  "error out" <- w8
  "Cases to go" <- w4
  "Station Selected" <- w2
